vi "Image from TRF Display.vi"(8 "Image Center X":i32, 9 "No Image File":path=path "\\\\acad1\\physics/Jurchescu-group/JW-PD/Mega Awesome/Image Not Found.png", 10 "Image Folder":path, 11 "Transfer File":path) -> (0 "Image Preview":T1(plugin-control), 1 "Image Out":T1(plugin-control), 2 "Image File":path=path "D:/UserData/Desktop/Jeremy/WFU/Research/Programs/VI mods/Image Not Found.png", 3 "Image Name":string, 4 "ROI File":path=path "D:/UserData/Desktop/Jeremy/WFU/Research/Programs/VI mods/Image Not Found.png")   [LabVIEW 2012]
uses:
  <vilib>/Utility/file.llb/Read From Spreadsheet File (string).vi
  <vilib>/regexp/Match Regular Expression.xnode
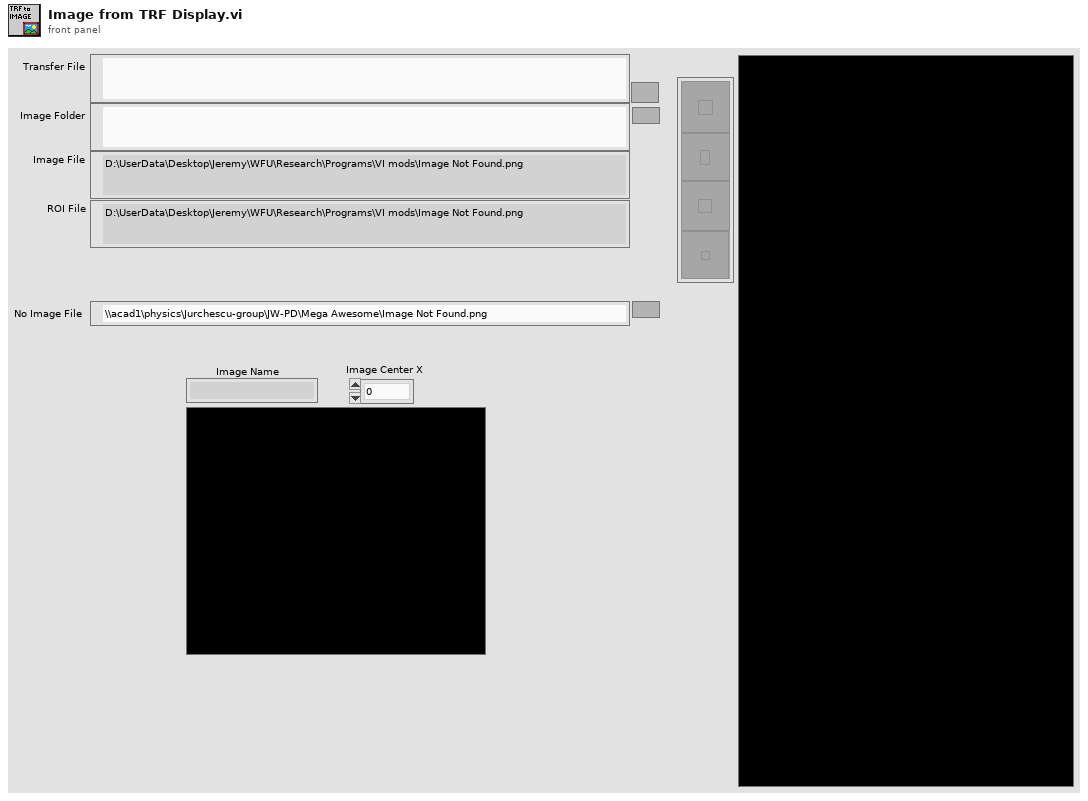
[diagram p1: front panel]
types:
  T1 = typedef "IMAQ Image.ctl" = refnum<image>
  T2 = cluster{"Global Rectangle":i32[], "Contours":cluster{"Contour Type":u32, "ROI Type":u32, "Points":i32[]}[]}
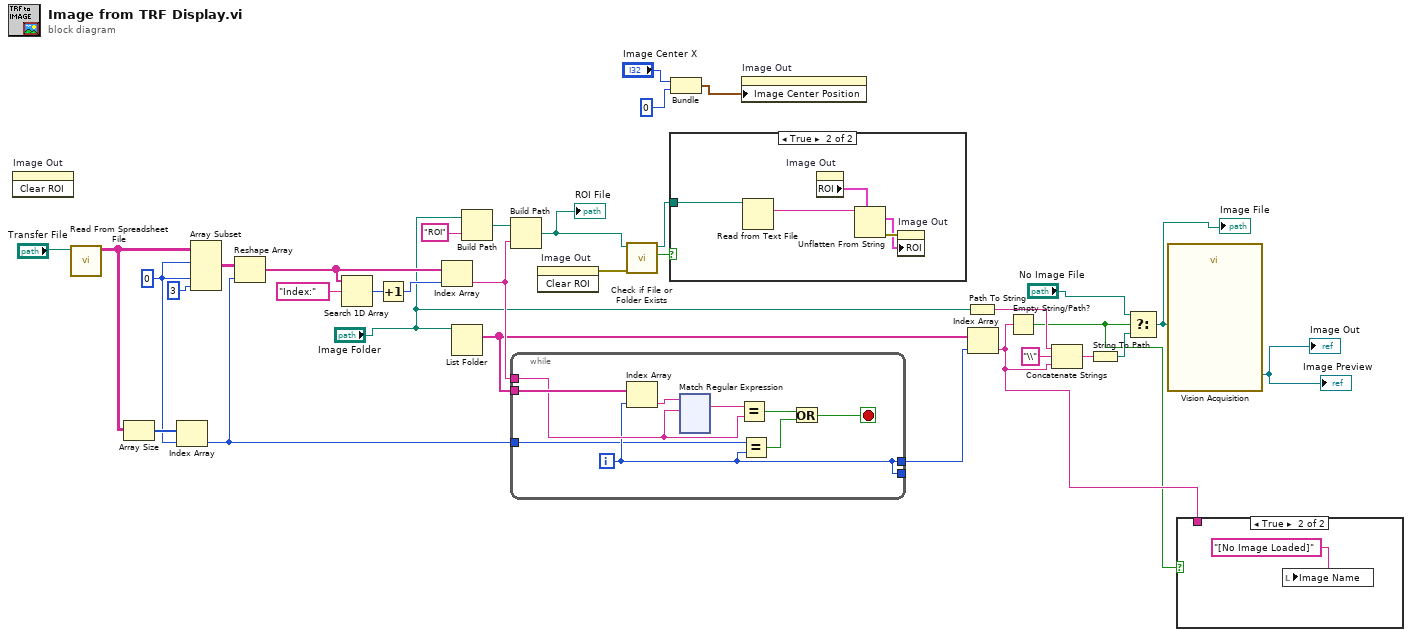
[diagram p0: block diagram]
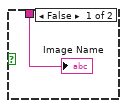
[diagram p2: hidden frame]
diagram:
  w22 = 0
  n1 = invoke on="Image Out" class="ImageControl" method="Clear ROI"() -> ()  [unwired: 3 in, 3 out]
  n2 = call-poly <vilib>:"Read From Spreadsheet File.vi"("file path (dialog if empty)"="Transfer File") -> ("all rows"=w24:string[][])  [unwired: 6 in, 4 out]
  n3 = Array Size(array=w24) -> (size(s)=w23:i32[])
  n4 = Index Array(array=w23, index=w22) -> (element=w16:i32)
  n5 = Array Subset(array=w24, index (row)=w22, index (col)=w22, length (col)=3) -> (w25:string[][])  [unwired: 1 in]
  n6 = Reshape Array(w25, w16) -> (w12:string[])
  n7 = Search 1D Array(1D array=w12, element="Index:") -> (index of element=w19:i32)  [unwired: 1 in]
  n8 = Increment(x=w19) -> (x+1=w20:i32)
  n9 = Index Array(array=w12, index=w20) -> (element=w33:string)
  n10 = List Folder(path="Image Folder") -> (filenames=w18:string[])  [unwired: 3 in, 3 out]
  n11 = Build Path(base path="Image Folder", name or relative path="ROI") -> (appended path=w32:path)
  n12 = Build Path(base path=w32, name or relative path=w33) -> (appended path=w6:path)
  "ROI File" <- w6
  n13 = while {
    tunnel: w18 -> [w41]
    tunnel: w33 -> [w39]
    tunnel: [w38] -> _
    tunnel: [w38] -> w17
    tunnel: w16 -> [w37]
    i -> [w38]
    stop <- w34 stop-if-true
    n14 = Index Array(array=w41, index=w38) -> (element=w42:string)
    n15 = xnode "Match Regular Expression"("input string"=w42, "regular expression"=w39) -> ("whole match"=w40:string)  [unwired: 4 in, 4 out]
    n16 = Equal?(x=w40, y=w39) -> (x = y?=w36:bool)
    n17 = Equal?(x=w37, y=w38) -> (x = y?=w35:bool)
    n18 = Or(x=w36, y=w35) -> (x .or. y?=w34:bool)
  }
  n19 = invoke on="Image Out" class="ImageControl" method="Clear ROI"() -> (error out=w28:errorcluster)  [unwired: 3 in, 2 out]
  n20 = call <vilib>:"Check if File or Folder Exists.vi"("error in (no error)"=w28, "path"=w6) -> ("file or folder exists?"=w30:bool, "dup path"=w29:path)  [unwired: 7 in, 1 out]
  n21 = case shown="True" w30 {
    tunnel: w29 -> [_ w154]
    frame False {
    }
    frame True {
      n22 = Read from Text File(file (use dialog)=w154) -> (text=w158:string)  [unwired: 3 in, 3 out]
      n23 = property on="Image Out" class="ImageControl"() -> ("ROI"=w155:T2)  [unwired: 2 in, 2 out]
      n24 = Unflatten From String(type=w155, binary string=w158) -> (value=w156:T2, error out=w157:errorcluster)  [unwired: 3 in, 1 out]
      n25 = property on="Image Out" class="ImageControl"(error in=w157, "ROI"=w156) -> ()  [unwired: 1 in, 2 out]
    }
  }
  n26 = Bundle("Image Center X"="Image Center X", 0) -> (w3:cluster{"Image Center X":i32, i32})  [unwired: 1 in]
  n27 = property on="Image Out" class="ImageControl"("Image Center Position"=w3) -> ()  [unwired: 2 in, 2 out]
  n28 = Path To String(path="Image Folder") -> (string=w15:string)
  n29 = Index Array(array=w18, index=w17) -> (element=w2:string)
  n30 = Empty String/Path?(string/path=w2) -> (empty?=w1:bool)
  n31 = Concatenate Strings(w15, "\\", w2) -> (w14:string)
  n32 = String To Path(string=w14) -> (path=w27:path)
  n33 = Select(t="No Image File", s=w1, f=w27) -> (s? t:f=w9:path)
  "Image File" <- w9
  n34 = call "Vision Acquisition"("Image Path"=w9) -> ("Image Out"=→"Image Out" →"Image Preview":T1)  [unwired: 25 in, 1 out]
  n35 = case shown="True" w1 {
    tunnel: w2 -> [w159 _]
    frame False {
      "Image Name" <- w159
    }
    frame True {
      n36 = local write "Image Name"("[No Image Loaded]") -> ()
    }
  }
